vi "Multi-tone Generator.vi"(0 "tone.parameters":T3(array[cluster])=[{"frequency"=0.0, "gain"=0.0, "phase"=0.0, "offset"={"offset I"=0.0, "offset Q"=0.0}}, {"frequency"=0.0, "gain"=0.0, "phase"=0.0, "offset"={"offset I"=0.0, "offset Q"=0.0}}] {"offset"."offset Q" format="%#.18g"; "offset"."offset I" format="%#.18g"}, 1 "tone.reset":bool, 7 "tone routing":cluster{"I":T1, "Q":T1}, 9 "input valid":bool=TRUE) -> (4 "tone data":T2[](array[typedef]), 10 "output valid":bool)   [LabVIEW 2019]
uses:
  <instrlib>/_niInstr/DSP/v1/Shared/Public/IQ Data.ctl
  Channel Control.ctl
  <instrlib>/_niInstr/DSP/v1/FPGA/Public/Sub VIs/Frequency Shift/Frequency Shift - 16 spc.vi
  <instrlib>/_niInstr/DSP/v1/FPGA/Public/Sub VIs/Digital Offset/Digital Offset - 1 spc.vi
  <instrlib>/_niInstr/DSP/v1/Xnodes/Public/Digital Offset/niInstr DSP v1 Digital Offset FPGA.xnode
  <instrlib>/_niInstr/DSP/v1/Shared/Public/IQ Offset.ctl
  <instrlib>/_niInstr/DSP/v1/Shared/niInstr DSP v1 Shared.lvlib
  <instrlib>/_niInstr/DSP/v1/FPGA/niInstr DSP v1 FPGA.lvlib
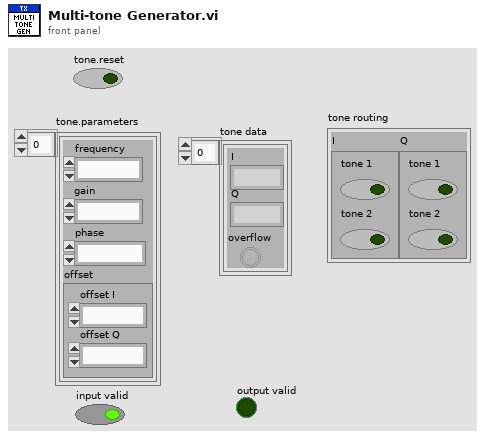
[diagram p1: front panel]
types:
  T1 = typedef "Channel Control.ctl" = cluster{"tone 1":bool, "tone 2":bool}
  T2 = typedef "niInstr DSP v1 Shared.lvlib/IQ Data.ctl" = cluster{"I":fxp<+/-,18,1>, "Q":fxp<+/-,18,1>, "overflow":bool}
  T3 = cluster{"frequency":fxp<+/-,48,0>, "gain":fxp<+/-,18,1>, "phase":fxp<+/-,21,0>, "offset":cluster{"offset I":fxp<+/-,18,1>, "offset Q":fxp<+/-,18,1>}}[]
  T4 = cluster{"frequency":fxp<+/-,48,0>, "gain":fxp<+/-,18,1>, "phase":fxp<+/-,21,0>, "offset":cluster{"offset I":fxp<+/-,18,1>, "offset Q":fxp<+/-,18,1>}}
  T5 = cluster{"offset I":fxp<+/-,18,1>, "offset Q":fxp<+/-,18,1>}
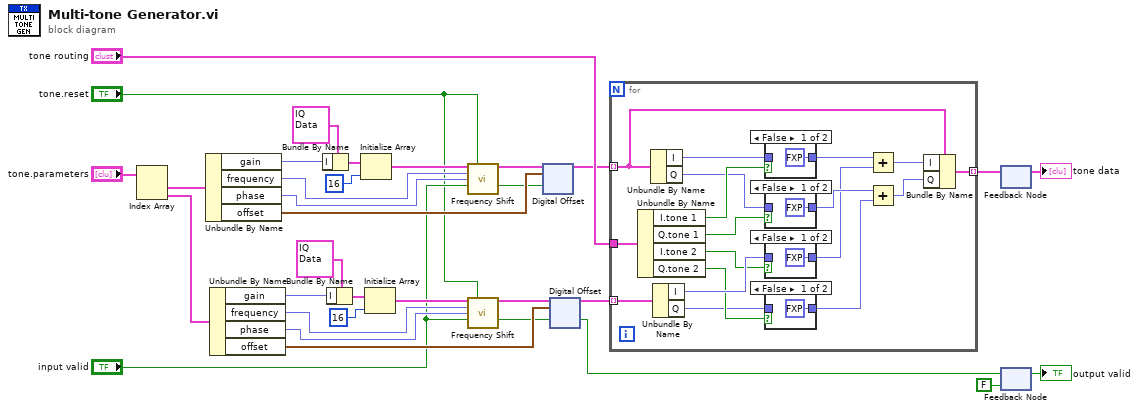
[diagram p0: block diagram]
diagram:
  n1 = Index Array(array="tone.parameters") -> (element #1=w22:T4, element #2=w21:T4)  [unwired: 2 in]
  n2 = Unbundle By Name(w22) -> ("gain"=w30:fxp<+/-,18,1>, "frequency"=w14:fxp<+/-,48,0>, "phase"=w13:fxp<+/-,21,0>, "offset"=w29:T5)
  n3 = Unbundle By Name(w21) -> ("gain"=w27:fxp<+/-,18,1>, "frequency"=w6:fxp<+/-,48,0>, "phase"=w5:fxp<+/-,21,0>, "offset"=w28:T5)
  n4 = Bundle By Name(cluster=T2 {"I"=0.0, "Q"=0.0, "overflow"=FALSE} ("tone.gain"), "I"=w30) -> (w31:T2)
  n5 = Bundle By Name(cluster=T2 {"I"=0.0, "Q"=0.0, "overflow"=FALSE} ("tone.gain"), "I"=w27) -> (w26:T2)
  n6 = Initialize Array(w31, 16 ("dimension size")) -> (w15:T2[])
  n7 = Initialize Array(w26, 16 ("dimension size")) -> (w10:T2[])
  n8 = call-poly <instrlib>:"Frequency Shift.vi"("data in"=w15, "reset"="tone.reset", "frequency shift"=w14, "phase"=w13, "input valid"="input valid") -> ("data out"=w1:T2[], "output valid"=w12:bool)  [unwired: 7 in, 2 out]
  n9 = call-poly <instrlib>:"Frequency Shift.vi"("data in"=w10, "reset"="tone.reset", "frequency shift"=w6, "phase"=w5, "input valid"="input valid") -> ("data out"=w9:T2[], "output valid"=w3:bool)  [unwired: 7 in, 2 out]
  n10 = xnode "Digital Offset"("data in"=w1, "offset"=w29, "input valid"=w12) -> ("data out"=w11:T2[])  [unwired: 2 in, 2 out]
  n11 = xnode "Digital Offset"("data in"=w9, "offset"=w28, "input valid"=w3) -> ("data out"=w7:T2[], "output valid"=w8:bool)  [unwired: 2 in, 1 out]
  n12 = for {
    tunnel: w11 -> [w49] mode=indexing
    tunnel: w7 -> [w51] mode=indexing
    tunnel: [w47] -> w20 mode=indexing
    tunnel: "tone routing" -> [w46]
    n13 = Unbundle By Name(w46) -> ("I.tone 1"=w45:bool, "Q.tone 1"=w41:bool, "I.tone 2"=w38:bool, "Q.tone 2"=w35:bool)
    n14 = Unbundle By Name(w49) -> ("I"=w44:fxp<+/-,18,1>, "Q"=w42:fxp<+/-,18,1>)
    n15 = Unbundle By Name(w51) -> ("I"=w39:fxp<+/-,18,1>, "Q"=w34:fxp<+/-,18,1>)
    n16 = case shown="False" w45 {
      tunnel: w44 -> [_ w59]
      tunnel: [fxp<+/-,18,1> 0.0 ("I") w59] -> w43
      frame False {
      }
      frame True {
      }
    }
    n17 = case shown="False" w41 {
      tunnel: w42 -> [_ w57]
      tunnel: [fxp<+/-,18,1> 0.0 ("I") w57] -> w40
      frame False {
      }
      frame True {
      }
    }
    n18 = case shown="False" w38 {
      tunnel: w39 -> [_ w55]
      tunnel: [fxp<+/-,18,1> 0.0 ("I") w55] -> w37
      frame False {
      }
      frame True {
      }
    }
    n19 = case shown="False" w35 {
      tunnel: w34 -> [_ w53]
      tunnel: [fxp<+/-,18,1> 0.0 ("I") w53] -> w36
      frame False {
      }
      frame True {
      }
    }
    n20 = Add(x=w43, y=w37) -> (x+y=w50:fxp<+/-,18,1>)
    n21 = Add(x=w40, y=w36) -> (x+y=w48:fxp<+/-,18,1>)
    n22 = Bundle By Name(cluster=w49, "I"=w50, "Q"=w48) -> (w47:T2)
  }
  n23 = feedback-in #1(w20) -> ()
  n24 = feedback #1() -> (→"tone data":T2[])  [unwired: 1 in]
  n25 = feedback #2(FALSE ("output valid")) -> (→"output valid":bool)
  n26 = feedback-in #2(w8) -> ()
